vi "daq.vi"() -> ()   [LabVIEW 2015]
uses:
  <vilib>/DAQmx/read.llb/DAQmx Read (Analog 1D Wfm NChan NSamp).vi
  <vilib>/DAQmx/create/channels.llb/DAQmx Create Channel (AI-Voltage-Basic).vi
  <vilib>/DAQmx/configure/timing.llb/DAQmx Timing (Sample Clock).vi
  <vilib>/DAQmx/miscellaneous.llb/DAQmx Fill In Error Info.vi
panel:
  out "Waveform Graph 2":dynamicdata(graph)
  out "Waveform Graph":dynamicdata(graph)
  out "error out":errorcluster
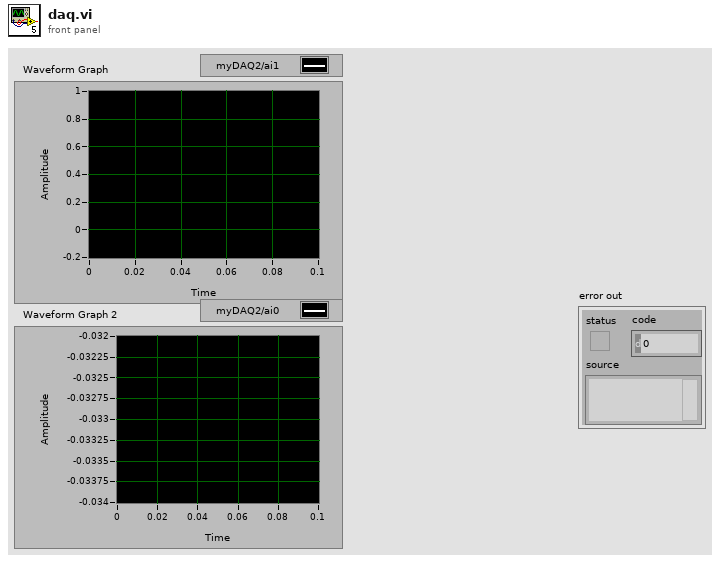
[diagram p1: front panel]
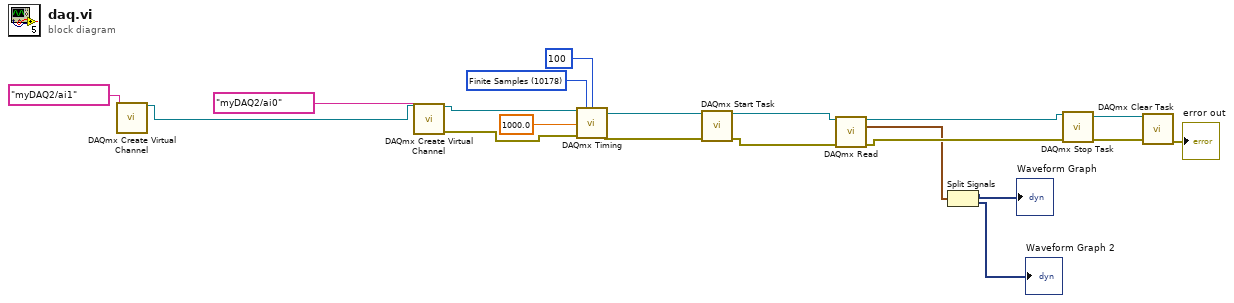
[diagram p0: block diagram]
diagram:
  w17 = 10178 items=["Finite Samples"=10178, "Continuous Samples"=10123, "Hardware Timed Single Point"=12522] ("sample mode")
  n1 = call-poly <vilib>:"DAQmx Create Virtual Channel.vi"("physical channels"=tag "myDAQ2/ai1") -> ("task out"=w4:refnum<k21>)  [unwired: 13 in, 1 out]
  n2 = call-poly <vilib>:"DAQmx Create Virtual Channel.vi"("task in"=w4, "physical channels"=tag "myDAQ2/ai0") -> ("task out"=w19:refnum<k21>, "error out"=w11:errorcluster)  [unwired: 12 in]
  n3 = call-poly <vilib>:"DAQmx Timing.vi"("task/channels in"=w19, "sample mode"=w17, "samples per channel"=100, "rate"=1000.0, "error in"=w11) -> ("task out"=w15:refnum<k21>, "error out"=w10:errorcluster)  [unwired: 9 in]
  n4 = call <vilib>:"DAQmx Start Task.vi"("task/channels in"=w15, "error in"=w10) -> ("task out"=w14:refnum<k21>, "error out"=w9:errorcluster)  [unwired: 12 in]
  n5 = call-poly <vilib>:"DAQmx Read.vi"("task/channels in"=w14, "error in"=w9) -> ("task out"=w13:refnum<k21>, "data"=w3:waveform(dbl)[], "error out"=w8:errorcluster)  [unwired: 11 in]
  n6 = Split Signals(w3) -> (→"Waveform Graph":dynamicdata, →"Waveform Graph 2":dynamicdata)  [unwired: 2 in]
  n7 = call <vilib>:"DAQmx Stop Task.vi"("task/channels in"=w13, "error in"=w8) -> ("task out"=w12:refnum<k21>, "error out"=w7:errorcluster)  [unwired: 12 in]
  n8 = call <vilib>:"DAQmx Clear Task.vi"("task in"=w12, "error in"=w7) -> ("error out"=→"error out":errorcluster)  [unwired: 13 in]
